vi "MGCC_StaEst_error_cal.vi"(8 "f_MGCC_StaEst_An":dbl[][](array[numeric]), 9 "f_MGCC_StaEst_Vn":dbl[][](array[numeric]), 10 "cluster":T1) -> ()   [LabVIEW 2016]
doc: "-----------------------------------------------------------------------------------------------------------------------\nCopyright <2019> <The University of Tennessee at Knoxville and the University of Tennessee Research Foundation>\nThis software is released under BSD-3 \nhttps://opensource.org/licenses/BSD-3-Clause \nAdditional license options available at https://utrf.tennessee.edu/industry/sample-agreements/\n-----------------------------------------------------------------------------------------------------------------------"
panel:
  out "Ang Err":dbl[][](array[numeric])
  out "Mag Err":dbl[][](array[numeric])
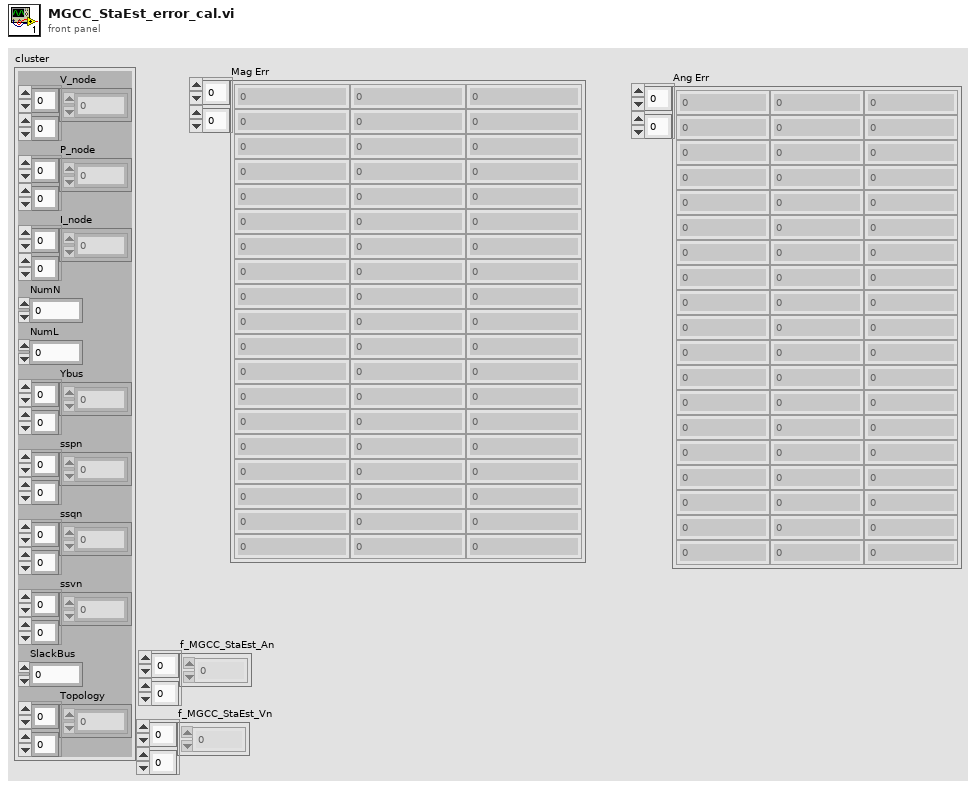
[diagram p1: front panel]
types:
  T1 = cluster{"V_node":cdb[][], "P_node":cdb[][], "I_node":cdb[][], "NumN":dbl, "NumL":dbl, "Ybus":cdb[][], "sspn":dbl[][], "ssqn":dbl[][], "ssvn":dbl[][], "SlackBus":dbl, "Topology":dbl[][]}
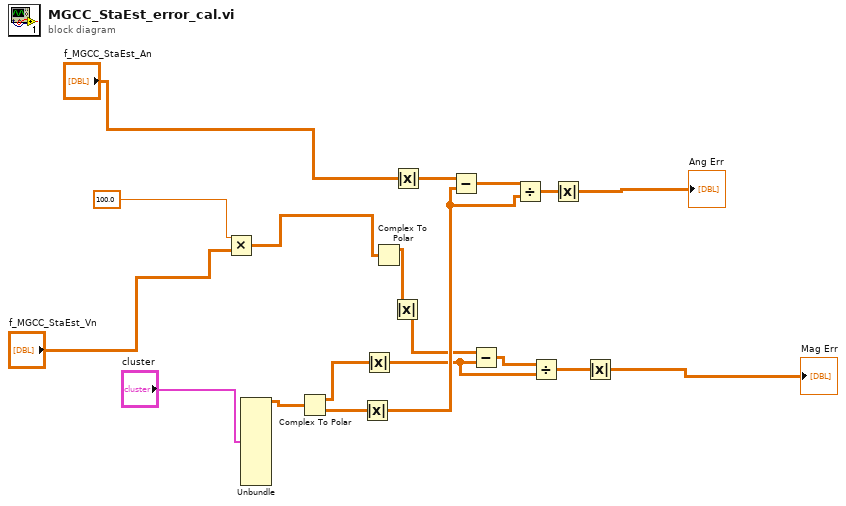
[diagram p0: block diagram]
diagram:
  n1 = Multiply(x=100.0, y="f_MGCC_StaEst_Vn") -> (x*y=w19:dbl[][])
  n2 = Unbundle("cluster") -> ("V_node"=w17:cdb[][])  [unwired: 10 out]
  n3 = Complex To Polar(r * e^(i*theta)=w17) -> (r=w14:dbl[][], theta=w11:dbl[][])
  n4 = Absolute Value(x=w11) -> (abs(x)=w8:dbl[][])
  n5 = Absolute Value(x=w14) -> (abs(x)=w6:dbl[][])
  n6 = Complex To Polar(r * e^(i*theta)=w19) -> (r=w16:dbl[][])  [unwired: 1 out]
  n7 = Absolute Value(x=w16) -> (abs(x)=w7:dbl[][])
  n8 = Absolute Value(x="f_MGCC_StaEst_An") -> (abs(x)=w9:dbl[][])
  n9 = Subtract(x=w9, y=w8) -> (x-y=w12:dbl[][])
  n10 = Subtract(x=w7, y=w6) -> (x-y=w15:dbl[][])
  n11 = Divide(x=w12, y=w8) -> (x/y=w10:dbl[][])
  n12 = Divide(x=w15, y=w6) -> (x/y=w13:dbl[][])
  n13 = Absolute Value(x=w10) -> (abs(x)=→"Ang Err":dbl[][])
  n14 = Absolute Value(x=w13) -> (abs(x)=→"Mag Err":dbl[][])
